vi "斜率与截距计算.vi"(10 "输入数值":u32) -> (2 "斜率与截距":T1)   [LabVIEW 2015]
uses:
  <vilib>/Utility/miscctls.llb/LVPointDoubleTypeDef.ctl
  Globle.vi
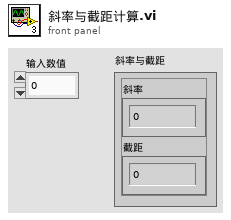
[diagram p1: front panel]
types:
  T1 = typedef "斜率与截距.ctl" = cluster{"斜率":dbl, "截距":dbl}
  T2 = typedef "LVPointDoubleTypeDef.ctl" = cluster{"X":dbl, "Y":dbl}
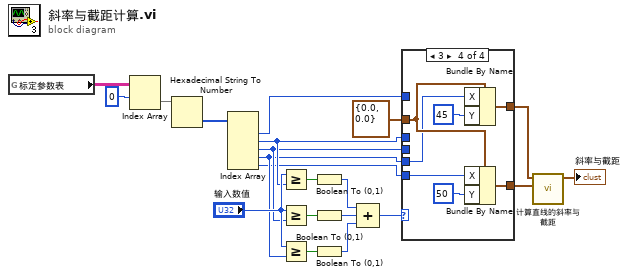
[diagram p0: block diagram]
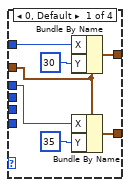
[diagram p2: hidden frame]
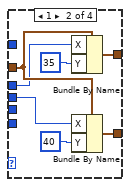
[diagram p3: hidden frame]
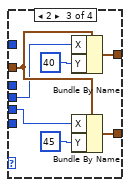
[diagram p4: hidden frame]
diagram:
  n1 = global read "Globle.vi" "标定参数表"() -> (w10:string[][])
  n2 = Index Array(array=w10, index (row)=0 ("禁用的索引 (列)")) -> (element=w12:string[])  [unwired: 1 in]
  n3 = Hexadecimal String To Number(string=w12) -> (number=w13:u32[])  [unwired: 2 in, 1 out]
  n4 = Index Array(array=w13) -> (element #1=w9:u32, element #2=w8:u32, element #3=w3:u32, element #4=w2:u32, element #5=w1:u32)  [unwired: 5 in]
  n5 = Greater Or Equal?(x="输入数值", y=w8) -> (x >= y?=w20:bool)
  n6 = Greater Or Equal?(x="输入数值", y=w3) -> (x >= y?=w18:bool)
  n7 = Greater Or Equal?(x="输入数值", y=w2) -> (x >= y?=w17:bool)
  n8 = Boolean To (0,1)(Boolean=w20) -> (0, 1=w19:i16)
  n9 = Boolean To (0,1)(Boolean=w18) -> (0, 1=w16:i16)
  n10 = Boolean To (0,1)(Boolean=w17) -> (0, 1=w15:i16)
  n11 = Compound Arithmetic op=ADD(w19, w16, w15) -> (w14:i16)
  n12 = case shown="3" w14 {
    tunnel: w9 -> [w28 _ _ _]
    tunnel: w8 -> [w26 w30 _ _]
    tunnel: [w24 w33 w40 w47] -> w7
    tunnel: [w23 w32 w39 w46] -> w6
    tunnel: T2 {"X"=0.0, "Y"=0.0} ("点A") -> [w22 w31 w38 w45]
    tunnel: w3 -> [_ w29 w37 _]
    tunnel: w2 -> [_ _ w36 w44]
    tunnel: w1 -> [_ _ _ w43]
    frame 0, Default {
      n13 = Bundle By Name(cluster=w22, "X"=w28, "Y"=30) -> (w24:T2)
      n14 = Bundle By Name(cluster=w22, "X"=w26, "Y"=35) -> (w23:T2)
    }
    frame 1 {
      n15 = Bundle By Name(cluster=w31, "X"=w30, "Y"=35) -> (w33:T2)
      n16 = Bundle By Name(cluster=w31, "X"=w29, "Y"=40) -> (w32:T2)
    }
    frame 2 {
      n17 = Bundle By Name(cluster=w38, "X"=w37, "Y"=40) -> (w40:T2)
      n18 = Bundle By Name(cluster=w38, "X"=w36, "Y"=45) -> (w39:T2)
    }
    frame 3 {
      n19 = Bundle By Name(cluster=w45, "X"=w44, "Y"=45) -> (w47:T2)
      n20 = Bundle By Name(cluster=w45, "X"=w43, "Y"=50) -> (w46:T2)
    }
  }
  n21 = call "计算直线的斜率与截距.vi"("点B"=w6, "点A"=w7) -> ("斜率与截距"=→"斜率与截距":T1)  [unwired: 8 in, 1 out]
